vi "Status Code.vi"(6 "LabPack Shared Library":path=path "", 8 "Error In":errorcluster, 11 "Status":T1) -> (0 "Error Out":errorcluster, 3 "Code":i32)   [LabVIEW 2018, in "Toolkit.lvlib"]
doc: "Converts a LabPack shared library status to an error code. Errors have a negative value, warnings have a positive value, and zero indicates an OK status."
uses:
  Toolkit.lvlib
  Controls/Status.ctl
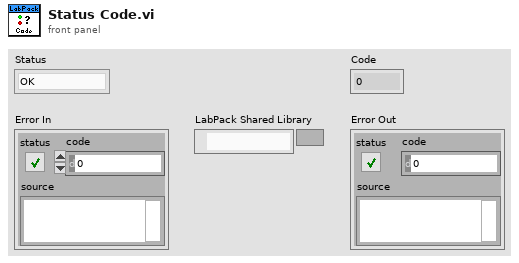
[diagram p1: front panel]
types:
  T1 = typedef "Toolkit.lvlib/Status.ctl" = enum32{"OK", "Out of Memory", "Null Value", "Encoder", "Decoder"}
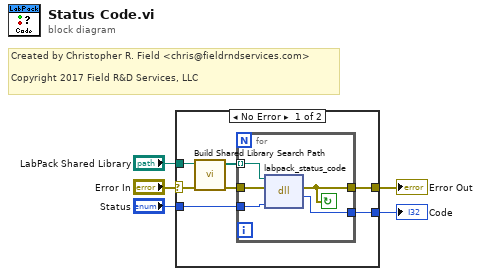
[diagram p0: block diagram]
diagram:
  # "Created by Christopher R. Field <chris@fieldrndservices.com>\n\nCopyright 2017 Field R&D Services, LLC"
  n1 = case shown="No Error" "Error In" {
    selector: "Error In" -> [w10 w18]
    tunnel: [w12 w18] -> w5
    tunnel: [w11 _] -> w3
    tunnel: "LabPack Shared Library" -> [w7 _]
    tunnel: "Status" -> [w6 _]
    frame No Error {
      n2 = call "Build Shared Library Search Path.vi"("Error In"=w10, "LabPack Shared Library"=w7) -> ("Error Out"=w9:errorcluster, "Search Path"=w8:path[])  [unwired: 8 in]
      n3 = for {
        tunnel: [w17] -> w11
        tunnel: w8 -> [w15] mode=indexing
        tunnel: w9 -> [w16]
        tunnel: [w14] -> w12
        tunnel: w6 -> [w13]
        stop <- w14 continue-if-true
        n4 = dll-call lib="D:/Users/cfield/Code/MessagePack/LabPack/LabVIEW/trunk/src/LabPack/Private/labpack-x64.dll" fn="labpack_status_code"(path in=w15, error in=w16, "status"=w13) -> (error out=w14:errorcluster, "return type"=w17:i32)  [unwired: 2 in, 1 out]
      }
    }
    frame Error {
    }
  }
  "Error Out" <- w5
  "Code" <- w3
